vi "DAQ.Sampling.Configure.vi"(8 "error in (no error)":errorcluster, 11 "Instrument.DAQ":refnum<class "Instrument.DAQ.lvclass">) -> (0 "error out":errorcluster, 2 "Sampling out":T1, 3 "Instrument.DAQ out":refnum<class "Instrument.DAQ.lvclass">)   [LabVIEW 2019, in "Instrument.DAQ.lvclass"]
uses:
  Instrument.DAQ.lvclass
  Typedefs/DAQ.Sampling.Sampling--Cluster.ctl
  Instrument.DAQ.lvclass/Instrument.DAQ.ctl
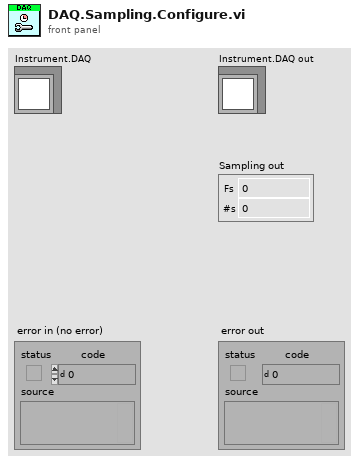
[diagram p1: front panel]
types:
  T1 = typedef "Instrument.DAQ.lvclass/DAQ.Sampling.Sampling--Cluster.ctl" = cluster{"Fs":dbl, "#s":i32}
  T2 = typedef "Instrument.DAQ.lvclass/DAQ.Sampling.Fs Mode--enum.ctl" = enum16{"Manual", "Auto Fs", "Max Fs"}
  T3 = typedef "Instrument.DAQ.lvclass/AO.Channel--Cluster--Array.ctl" = T4[]
  T4 = typedef "Instrument.DAQ.lvclass/AO.Channel--Cluster.ctl" = cluster{"Enable?":bool, "Channel":i32, "Amplitude":dbl, "Offset":dbl, "Frequency":dbl, "Phase":dbl, "Function":T5, "Sweeping?":bool}
  T5 = typedef "Instrument.DAQ.lvclass/AO.Channel.Function--Enum.ctl" = enum16{"Sine", "Triangle", "Square"}
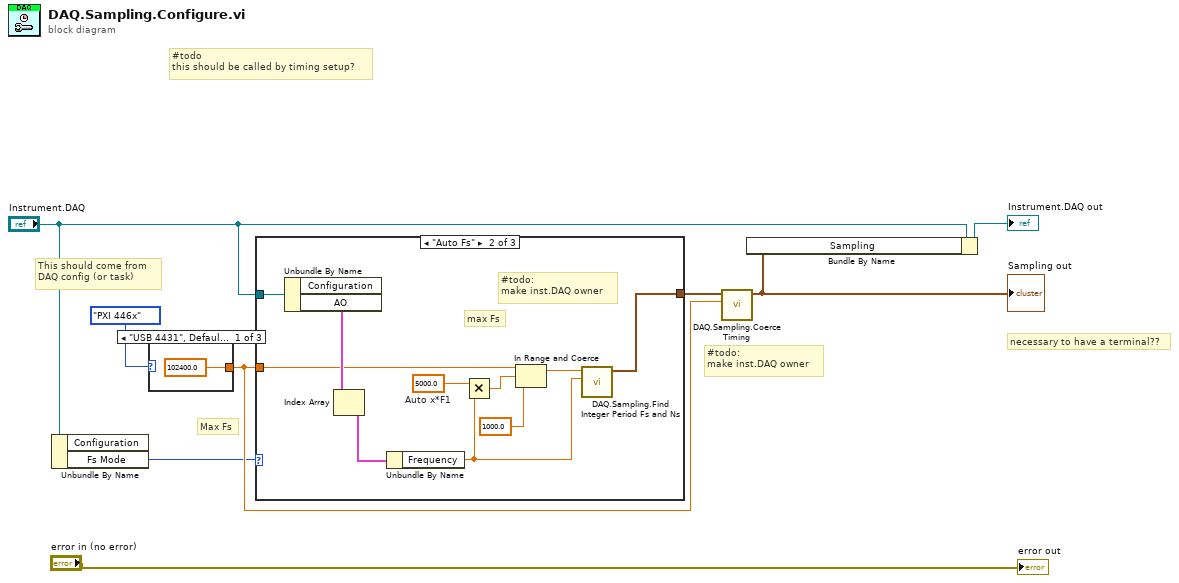
[diagram p0: block diagram]
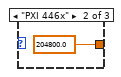
[diagram p2: hidden frame]
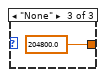
[diagram p3: hidden frame]
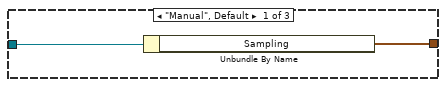
[diagram p4: hidden frame]
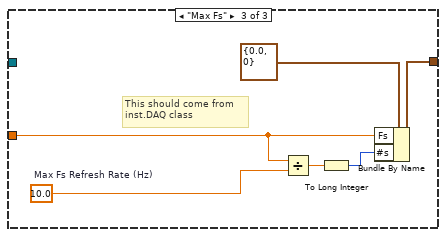
[diagram p5: hidden frame]
diagram:
  # "#todo\nthis should be called by timing setup?"
  # "necessary to have a terminal??"
  # "#todo:\nmake inst.DAQ owner"
  # "This should come from\nDAQ config (or task)"
  # "Max Fs"
  n1 = Unbundle By Name("Instrument.DAQ") -> ("Fs Mode"=w2:T2)  [unwired: 1 out]
  n2 = case shown="\"USB 4431\", Default" enum16{"None", "USB 4431", "PXI 446x"}."PXI 446x" ("DAQ Type") {
    tunnel: [102400.0 ("upper limit") 204800.0 ("upper limit") 204800.0 ("upper limit")] -> w7
    frame "USB 4431", Default {
    }
    frame "PXI 446x" {
    }
    frame "None" {
    }
  }
  n3 = case shown="\"Auto Fs\"" w2 {
    tunnel: [w12 w17 w24] -> w6
    tunnel: "Instrument.DAQ" -> [w13 w19 _]
    tunnel: w7 -> [_ w21 w29]
    frame "Manual", Default {
      n4 = Unbundle By Name(w13) -> ("Sampling"=w12:T1)
    }
    frame "Auto Fs" {
      w16 = 5000.0  # Auto x*F1
      # "#todo:\nmake inst.DAQ owner"
      # "max Fs"
      n5 = Unbundle By Name(w19) -> ("AO"=w22:T3)  [unwired: 1 out]
      n6 = Index Array(array=w22) -> (element=w14:T4)  [unwired: 1 in]
      n7 = Unbundle By Name(w14) -> ("Frequency"=w18:dbl)
      n8 = Multiply(x=w16, y=w18) -> (x*y=w20:dbl)
      n9 = In Range and Coerce(upper limit=w21, x=w20, lower limit=1000.0) -> (coerced(x)=w23:dbl)  [unwired: 1 out]
      n10 = call "DAQ.Sampling.Find Integer Period Fs and Ns.vi"("f integer"=w18, "Max Fs"=w23) -> ("Timing out"=w17:T1)  [unwired: 9 in]
    }
    frame "Max Fs" {
      w26 = 10.0  # Max Fs Refresh Rate (Hz)
      # "This should come from\ninst.DAQ class"
      n11 = Divide(x=w29, y=w26) -> (x/y=w28:dbl)
      n12 = To Long Integer(number=w28) -> (32bit integer=w27:i32)
      n13 = Bundle By Name(cluster=T1 {"Fs"=0.0, "#s"=0} ("Sampling out"), "Fs"=w29, "#s"=w27) -> (w24:T1)
    }
  }
  n14 = call "DAQ.Sampling.Coerce Timing.vi"("Max Fs"=w7, "Sampling in"=w6) -> ("Sampling out"=w5:T1)  [unwired: 9 in]
  "Sampling out" <- w5
  n15 = Bundle By Name(cluster="Instrument.DAQ", "Sampling"=w5) -> (→"Instrument.DAQ out":refnum<class "Instrument.DAQ.lvclass">)
  "error out" <- "error in (no error)"
